vi "Check If VI is Test Method.vi"(8 "error in (no error)":errorcluster, 11 "VI Name":string) -> (0 "error out":errorcluster, 3 "Is Test Method?":bool)   [LabVIEW 2020, in "Test Finder.lvclass"]
uses:
  Test Finder.lvclass
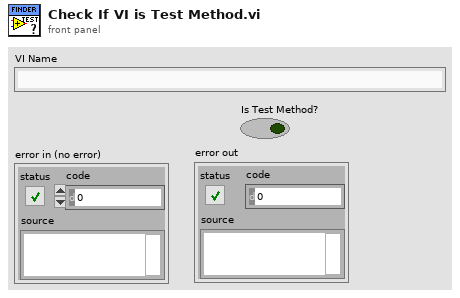
[diagram p1: front panel]
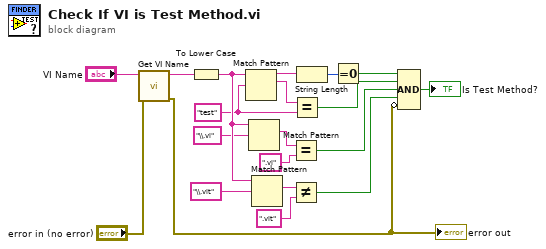
[diagram p0: block diagram]
diagram:
  w8 = "test" ("regular expression")
  n1 = call "Get VI Name.vi"("error in (no error)"="error in (no error)", "Fully Qualified VI name"="VI Name") -> ("error out"=w3:errorcluster, "VI Name"=w5:string)  [unwired: 8 in]
  "error out" <- w3
  n2 = To Lower Case(string=w5) -> (all lower case string=w16:string)
  n3 = Match Pattern(string=w16, regular expression=w8) -> (before substring=w9:string, match substring=w7:string)  [unwired: 1 in, 2 out]
  n4 = Match Pattern(string=w16, regular expression="\\.vi") -> (match substring=w13:string)  [unwired: 1 in, 3 out]
  n5 = Match Pattern(string=w16, regular expression="\\.vit") -> (match substring=w17:string)  [unwired: 1 in, 3 out]
  n6 = Equal?(x=w13, y=".vi") -> (x = y?=w15:bool)
  n7 = Not Equal?(x=w17, y=".vit") -> (x != y?=w19:bool)
  n8 = Equal?(x=w7, y=w8) -> (x = y?=w12:bool)
  n9 = String Length(string=w9) -> (length=w10:i32)
  n10 = Equal To 0?(x=w10) -> (x = 0?=w11:bool)
  n11 = Compound Arithmetic op=AND(w11, w12, w15, w19, invert w3) -> (→"Is Test Method?":bool)
